vi "Setup For Triggered Images USB3 v4.4.vi"(5 "error in":errorcluster caption="error in (no error)", 6 "Timeout":u32=20000, 7 "Gain":dbl, 8 "Shutter speed":dbl=30000.0, 9 "Camera Name":T3="FL3-32S2M") -> (0 "Error out":errorcluster caption="error in (no error)", 1 "Session Out":T3="FL3-32S2M", 2 "Height":u32=1552, 3 "Width":u32=2080, 4 "DeviceID":string="FL3-32S2M")   [LabVIEW 2013]
doc: "The Grab and Attributes Setup VI acquires images continuously and displays the images in an image control using high-level acquisition VIs. The VI also modifes the camera attributes while acquiring images. A grab is appropriate for high-speed applications in which you need to process only one image at a time."
uses:
  <vilib>/userdefined/High Color/IMAQdx.ctl
  <vilib>/vision/driver/IMAQdx.llb/IMAQdx Attribute Type.ctl
  <vilib>/vision/driver/IMAQdx.llb/IMAQdx Attribute Visibility.ctl
  <vilib>/vision/driver/NI_Vision_Acquisition_Software.lvlib
  <resource>/objmgr/imaqdx.rc
panel:
  in  "stop":bool
  out "Attribute Information Array":T2(array[cluster])=[{"Attribute Type"=enum."U32", "Readable"=TRUE, "Writable"=TRUE, "Attribute Name"="AcquisitionAttributes::AdvancedGenicam::CommandTimeout"}, {"Attribute Type"=enum."U32", "Readable"=TRUE, "Writable"=TRUE, "Attribute Name"="AcquisitionAttributes::AdvancedGenicam::EventQueueDepth"}, {"Attribute Type"=enum."Bool", "Readable"=TRUE, "Writable"=FALSE, "Attribute Name"="AcquisitionAttributes::AdvancedGenicam::EventsEnabled"}, {"Attribute Type"=enum."Bool", "Readable"=TRUE, "Writable"=FALSE, "Attribute Name"="AcquisitionAttributes::AdvancedGenicam::EventsSupported"}, {"Attribute Type"=enum."Bool", "Readable"=TRUE, "Writable"=TRUE, "Attribute Name"="AcquisitionAttributes::AdvancedGenicam::IgnoreCameraValidationErrors"}, {"Attribute Type"=enum."U32", "Readable"=TRUE, "Writable"=FALSE, "Attribute Name"="AcquisitionAttributes::AdvancedUSB3Vision::ActualMaximumPayloadTransferSize"}, {"Attribute Type"=enum."U32", "Readable"=TRUE, "Writable"=FALSE, "Attribute Name"="AcquisitionAttributes::AdvancedUSB3Vision::RequiredPayloadSizeAlignment"}, {"Attribute Type"=enum."Enum", "Readable"=TRUE, "Writable"=TRUE, "Attribute Name"="AcquisitionAttributes::Bayer::Algorithm"}, {"Attribute Type"=enum."DBL", "Readable"=TRUE, "Writable"=TRUE, "Attribute Name"="AcquisitionAttributes::Bayer::GainB"}, {"Attribute Type"=enum."DBL", "Readable"=TRUE, "Writable"=TRUE, "Attribute Name"="AcquisitionAttributes::Bayer::GainG"}, {"Attribute Type"=enum."DBL", "Readable"=TRUE, "Writable"=TRUE, "Attribute Name"="AcquisitionAttributes::Bayer::GainR"}, {"Attribute Type"=enum."Enum", "Readable"=TRUE, "Writable"=TRUE, "Attribute Name"="AcquisitionAttributes::Bayer::Pattern"}, {"Attribute Type"=enum."Bool", "Readable"=TRUE, "Writable"=TRUE, "Attribute Name"="AcquisitionAttributes::ChunkDataDecoding::ChunkDataDecodingEnabled"}, {"Attribute Type"=enum."U32", "Readable"=TRUE, "Writable"=TRUE, "Attribute Name"="AcquisitionAttributes::ChunkDataDecoding::MaximumChunkCopySize"}, {"Attribute Type"=enum."Enum", "Readable"=TRUE, "Writable"=TRUE, "Attribute Name"="CameraAttributes::AnalogControl::GainAuto"}, {"Attribute Type"=enum."DBL", "Readable"=TRUE, "Writable"=TRUE, "Attribute Name"="CameraAttributes::AnalogControl::Gain"}, {"Attribute Type"=enum."DBL", "Readable"=TRUE, "Writable"=FALSE, "Attribute Name"="CameraAttributes::AnalogControl::AutoGainLowerLimit"}, {"Attribute Type"=enum."DBL", "Readable"=TRUE, "Writable"=FALSE, "Attribute Name"="CameraAttributes::AnalogControl::AutoGainUpperLimit"}, {"Attribute Type"=enum."DBL", "Readable"=TRUE, "Writable"=TRUE, "Attribute Name"="CameraAttributes::AnalogControl::BlackLevel"}, {"Attribute Type"=enum."Bool", "Readable"=TRUE, "Writable"=TRUE, "Attribute Name"="CameraAttributes::AnalogControl::BlackLevelEnabled"}, {"Attribute Type"=enum."DBL", "Readable"=TRUE, "Writable"=FALSE, "Attribute Name"="CameraAttributes::AnalogControl::Gamma"}, {"Attribute Type"=enum."Bool", "Readable"=TRUE, "Writable"=TRUE, "Attribute Name"="CameraAttributes::AnalogControl::GammaEnabled"}, {"Attribute Type"=enum."I64", "Readable"=TRUE, "Writable"=FALSE, "Attribute Name"="CameraAttributes::AnalogControl::Sharpness"}, {"Attribute Type"=enum."Bool", "Readable"=TRUE, "Writable"=TRUE, "Attribute Name"="CameraAttributes::AnalogControl::SharpnessEnabled"}, {"Attribute Type"=enum."Enum", "Readable"=TRUE, "Writable"=FALSE, "Attribute Name"="CameraAttributes::AnalogControl::SharpnessAuto"}, {"Attribute Type"=enum."Bool", "Readable"=FALSE, "Writable"=FALSE, "Attribute Name"="CameraAttributes::AnalogControl::HueEnabled"}, {"Attribute Type"=enum."Bool", "Readable"=FALSE, "Writable"=FALSE, "Attribute Name"="CameraAttributes::AnalogControl::SaturationEnabled"}, {"Attribute Type"=enum."String", "Readable"=TRUE, "Writable"=FALSE, "Attribute Name"="CameraAttributes::DeviceControl::DeviceVendorName"}, {"Attribute Type"=enum."String", "Readable"=TRUE, "Writable"=FALSE, "Attribute Name"="CameraAttributes::DeviceControl::DeviceModelName"}, {"Attribute Type"=enum."String", "Readable"=TRUE, "Writable"=FALSE, "Attribute Name"="CameraAttributes::DeviceControl::DeviceFamilyName"}, {"Attribute Type"=enum."String", "Readable"=TRUE, "Writable"=FALSE, "Attribute Name"="CameraAttributes::DeviceControl::DeviceVersion"}, {"Attribute Type"=enum."String", "Readable"=TRUE, "Writable"=FALSE, "Attribute Name"="CameraAttributes::DeviceControl::DeviceSVNVersion"}, {"Attribute Type"=enum."String", "Readable"=TRUE, "Writable"=FALSE, "Attribute Name"="CameraAttributes::DeviceControl::DeviceID"}, {"Attribute Type"=enum."String", "Readable"=TRUE, "Writable"=TRUE, "Attribute Name"="CameraAttributes::DeviceControl::DeviceUserID"}, {"Attribute Type"=enum."Enum", "Readable"=TRUE, "Writable"=FALSE, "Attribute Name"="CameraAttributes::DeviceControl::DeviceScanType"}, {"Attribute Type"=enum."DBL", "Readable"=TRUE, "Writable"=FALSE, "Attribute Name"="CameraAttributes::DeviceControl::DeviceTemperature"}, {"Attribute Type"=enum."I64", "Readable"=TRUE, "Writable"=FALSE, "Attribute Name"="CameraAttributes::DeviceControl::U3VDeviceCapability"}, {"Attribute Type"=enum."Bool", "Readable"=TRUE, "Writable"=FALSE, "Attribute Name"="CameraAttributes::DeviceControl::UserNameAvailable"}, {"Attribute Type"=enum."Bool", "Readable"=TRUE, "Writable"=FALSE, "Attribute Name"="CameraAttributes::DeviceControl::AccessPrivilegeAvailable"}, {"Attribute Type"=enum."Bool", "Readable"=TRUE, "Writable"=FALSE, "Attribute Name"="CameraAttributes::DeviceControl::MessageChannelSupported"}, {"Attribute Type"=enum."Bool", "Readable"=TRUE, "Writable"=FALSE, "Attribute Name"="CameraAttributes::DeviceControl::TimestampSupported"}, {"Attribute Type"=enum."I64", "Readable"=TRUE, "Writable"=FALSE, "Attribute Name"="CameraAttributes::DeviceControl::StringEncoding"}, {"Attribute Type"=enum."Bool", "Readable"=TRUE, "Writable"=FALSE, "Attribute Name"="CameraAttributes::DeviceControl::FamilyRegisterAvailable"}, {"Attribute Type"=enum."Bool", "Readable"=TRUE, "Writable"=FALSE, "Attribute Name"="CameraAttributes::DeviceControl::SBRMSupported"}, {"Attribute Type"=enum."Bool", "Readable"=TRUE, "Writable"=FALSE, "Attribute Name"="CameraAttributes::DeviceControl::EndianessRegistersSupported"}, {"Attribute Type"=enum."Bool", "Readable"=TRUE, "Writable"=FALSE, "Attribute Name"="CameraAttributes::DeviceControl::WrittenLengthFieldSupported"}, {"Attribute Type"=enum."I64", "Readable"=TRUE, "Writable"=FALSE, "Attribute Name"="CameraAttributes::DeviceControl::DeviceMaxThroughput"}, {"Attribute Type"=enum."I64", "Readable"=TRUE, "Writable"=TRUE, "Attribute Name"="CameraAttributes::DeviceControl::DeviceLinkThroughputLimit"}, {"Attribute Type"=enum."Enum", "Readable"=TRUE, "Writable"=TRUE, "Attribute Name"="CameraAttributes::AcquisitionControl::TriggerSelector"}, {"Attribute Type"=enum."Enum", "Readable"=TRUE, "Writable"=TRUE, "Attribute Name"="CameraAttributes::AcquisitionControl::TriggerMode"}, {"Attribute Type"=enum."Command", "Readable"=FALSE, "Writable"=FALSE, "Attribute Name"="CameraAttributes::AcquisitionControl::TriggerSoftware"}, {"Attribute Type"=enum."Enum", "Readable"=TRUE, "Writable"=TRUE, "Attribute Name"="CameraAttributes::AcquisitionControl::TriggerSource"}, {"Attribute Type"=enum."Enum", "Readable"=TRUE, "Writable"=TRUE, "Attribute Name"="CameraAttributes::AcquisitionControl::TriggerActivation"}, {"Attribute Type"=enum."DBL", "Readable"=TRUE, "Writable"=TRUE, "Attribute Name"="CameraAttributes::AcquisitionControl::TriggerDelay"}, {"Attribute Type"=enum."Bool", "Readable"=TRUE, "Writable"=TRUE, "Attribute Name"="CameraAttributes::AcquisitionControl::TriggerDelayEnabled"}, {"Attribute Type"=enum."Enum", "Readable"=TRUE, "Writable"=TRUE, "Attribute Name"="CameraAttributes::AcquisitionControl::ExposureMode"}, {"Attribute Type"=enum."Enum", "Readable"=TRUE, "Writable"=TRUE, "Attribute Name"="CameraAttributes::AcquisitionControl::ExposureAuto"}, {"Attribute Type"=enum."DBL", "Readable"=TRUE, "Writable"=FALSE, "Attribute Name"="CameraAttributes::AcquisitionControl::ExposureTime"}, {"Attribute Type"=enum."DBL", "Readable"=TRUE, "Writable"=TRUE, "Attribute Name"="CameraAttributes::AcquisitionControl::AutoExposureTimeLowerLimit"}, {"Attribute Type"=enum."DBL", "Readable"=TRUE, "Writable"=TRUE, "Attribute Name"="CameraAttributes::AcquisitionControl::AutoExposureTimeUpperLimit"}, {"Attribute Type"=enum."Enum", "Readable"=TRUE, "Writable"=TRUE, "Attribute Name"="CameraAttributes::AcquisitionControl::AcquisitionMode"}, {"Attribute Type"=enum."Enum", "Readable"=TRUE, "Writable"=TRUE, "Attribute Name"="CameraAttributes::AcquisitionControl::AcquisitionFrameRateAuto"}, {"Attribute Type"=enum."Bool", "Readable"=TRUE, "Writable"=TRUE, "Attribute Name"="CameraAttributes::AcquisitionControl::AcquisitionFrameRateEnabled"}, {"Attribute Type"=enum."DBL", "Readable"=TRUE, "Writable"=FALSE, "Attribute Name"="CameraAttributes::AcquisitionControl::AcquisitionFrameRate"}, {"Attribute Type"=enum."I64", "Readable"=FALSE, "Writable"=FALSE, "Attribute Name"="CameraAttributes::AcquisitionControl::AcquisitionFrameCount"}, {"Attribute Type"=enum."Enum", "Readable"=TRUE, "Writable"=TRUE, "Attribute Name"="CameraAttributes::ImageFormatControl::PixelFormat"}, {"Attribute Type"=enum."I64", "Readable"=TRUE, "Writable"=TRUE, "Attribute Name"="CameraAttributes::ImageFormatControl::Width"}, {"Attribute Type"=enum."I64", "Readable"=TRUE, "Writable"=TRUE, "Attribute Name"="CameraAttributes::ImageFormatControl::Height"}, {"Attribute Type"=enum."I64", "Readable"=TRUE, "Writable"=TRUE, "Attribute Name"="CameraAttributes::ImageFormatControl::OffsetX"}, {"Attribute Type"=enum."I64", "Readable"=TRUE, "Writable"=TRUE, "Attribute Name"="CameraAttributes::ImageFormatControl::OffsetY"}, {"Attribute Type"=enum."I64", "Readable"=TRUE, "Writable"=FALSE, "Attribute Name"="CameraAttributes::ImageFormatControl::SensorWidth"}, {"Attribute Type"=enum."I64", "Readable"=TRUE, "Writable"=FALSE, "Attribute Name"="CameraAttributes::ImageFormatControl::SensorHeight"}, {"Attribute Type"=enum."I64", "Readable"=TRUE, "Writable"=FALSE, "Attribute Name"="CameraAttributes::ImageFormatControl::WidthMax"}, {"Attribute Type"=enum."I64", "Readable"=TRUE, "Writable"=FALSE, "Attribute Name"="CameraAttributes::ImageFormatControl::HeightMax"}, {"Attribute Type"=enum."Enum", "Readable"=TRUE, "Writable"=TRUE, "Attribute Name"="CameraAttributes::ImageFormatControl::VideoMode"}, {"Attribute Type"=enum."I64", "Readable"=TRUE, "Writable"=FALSE, "Attribute Name"="CameraAttributes::ImageFormatControl::BinningHorizontal"}, {"Attribute Type"=enum."I64", "Readable"=TRUE, "Writable"=TRUE, "Attribute Name"="CameraAttributes::ImageFormatControl::BinningVertical"}, {"Attribute Type"=enum."Bool", "Readable"=TRUE, "Writable"=TRUE, "Attribute Name"="CameraAttributes::ImageFormatControl::ReverseX"}, {"Attribute Type"=enum."Enum", "Readable"=TRUE, "Writable"=FALSE, "Attribute Name"="CameraAttributes::ImageFormatControl::PixelCoding"}, {"Attribute Type"=enum."Enum", "Readable"=TRUE, "Writable"=FALSE, "Attribute Name"="CameraAttributes::ImageFormatControl::PixelSize"}, {"Attribute Type"=enum."Enum", "Readable"=TRUE, "Writable"=FALSE, "Attribute Name"="CameraAttributes::ImageFormatControl::PixelColorFilter"}, {"Attribute Type"=enum."I64", "Readable"=TRUE, "Writable"=FALSE, "Attribute Name"="CameraAttributes::ImageFormatControl::PixelDynamicRangeMin"}, {"Attribute Type"=enum."I64", "Readable"=TRUE, "Writable"=FALSE, "Attribute Name"="CameraAttributes::ImageFormatControl::PixelDynamicRangeMax"}, {"Attribute Type"=enum."Enum", "Readable"=TRUE, "Writable"=TRUE, "Attribute Name"="CameraAttributes::ImageFormatControl::TestImageSelector"}, {"Attribute Type"=enum."I64", "Readable"=TRUE, "Writable"=FALSE, "Attribute Name"="CameraAttributes::UserSetControl::UserSetCurrent"}, {"Attribute Type"=enum."Enum", "Readable"=TRUE, "Writable"=TRUE, "Attribute Name"="CameraAttributes::UserSetControl::UserSetSelector"}, {"Attribute Type"=enum."Enum", "Readable"=TRUE, "Writable"=TRUE, "Attribute Name"="CameraAttributes::UserSetControl::UserSetDefaultSelector"}, {"Attribute Type"=enum."Command", "Readable"=FALSE, "Writable"=TRUE, "Attribute Name"="CameraAttributes::UserSetControl::UserSetLoad"}, {"Attribute Type"=enum."Command", "Readable"=FALSE, "Writable"=TRUE, "Attribute Name"="CameraAttributes::UserSetControl::UserSetSave"}, {"Attribute Type"=enum."Enum", "Readable"=TRUE, "Writable"=TRUE, "Attribute Name"="CameraAttributes::DigitalIOControl::LineSelector"}, {"Attribute Type"=enum."Enum", "Readable"=TRUE, "Writable"=TRUE, "Attribute Name"="CameraAttributes::DigitalIOControl::LineMode"}, {"Attribute Type"=enum."Enum", "Readable"=FALSE, "Writable"=FALSE, "Attribute Name"="CameraAttributes::DigitalIOControl::LineSource"}, {"Attribute Type"=enum."Bool", "Readable"=FALSE, "Writable"=FALSE, "Attribute Name"="CameraAttributes::DigitalIOControl::LineInverter"}, {"Attribute Type"=enum."I64", "Readable"=TRUE, "Writable"=TRUE, "Attribute Name"="CameraAttributes::DigitalIOControl::LineDebouncerTimeRaw"}, {"Attribute Type"=enum."Bool", "Readable"=TRUE, "Writable"=FALSE, "Attribute Name"="CameraAttributes::DigitalIOControl::LineStatus"}, {"Attribute Type"=enum."I64", "Readable"=TRUE, "Writable"=FALSE, "Attribute Name"="CameraAttributes::DigitalIOControl::LineStatusAll"}, {"Attribute Type"=enum."Bool", "Readable"=FALSE, "Writable"=FALSE, "Attribute Name"="CameraAttributes::DigitalIOControl::StrobeEnabled"}, {"Attribute Type"=enum."DBL", "Readable"=FALSE, "Writable"=FALSE, "Attribute Name"="CameraAttributes::DigitalIOControl::StrobeDelay"}, {"Attribute Type"=enum."DBL", "Readable"=FALSE, "Writable"=FALSE, "Attribute Name"="CameraAttributes::DigitalIOControl::StrobeDuration"}, {"Attribute Type"=enum."Bool", "Readable"=FALSE, "Writable"=FALSE, "Attribute Name"="CameraAttributes::DigitalIOControl::UserOutputValue"}, {"Attribute Type"=enum."I64", "Readable"=TRUE, "Writable"=FALSE, "Attribute Name"="CameraAttributes::TransportLayerControl::PayloadSize"}, {"Attribute Type"=enum."I64", "Readable"=TRUE, "Writable"=FALSE, "Attribute Name"="CameraAttributes::TransportLayerControl::GenCPVersionMajor"}, {"Attribute Type"=enum."I64", "Readable"=TRUE, "Writable"=FALSE, "Attribute Name"="CameraAttributes::TransportLayerControl::GenCPVersionMinor"}, {"Attribute Type"=enum."I64", "Readable"=TRUE, "Writable"=FALSE, "Attribute Name"="CameraAttributes::TransportLayerControl::U3VTimestamp"}, {"Attribute Type"=enum."Command", "Readable"=FALSE, "Writable"=TRUE, "Attribute Name"="CameraAttributes::TransportLayerControl::U3VTimestampLatch"}, {"Attribute Type"=enum."I64", "Readable"=TRUE, "Writable"=FALSE, "Attribute Name"="CameraAttributes::TransportLayerControl::U3VTimestampIncrement"}, {"Attribute Type"=enum."I64", "Readable"=TRUE, "Writable"=FALSE, "Attribute Name"="CameraAttributes::TransportLayerControl::U3VVersionMajor"}, {"Attribute Type"=enum."I64", "Readable"=TRUE, "Writable"=FALSE, "Attribute Name"="CameraAttributes::TransportLayerControl::U3VVersionMinor"}, {"Attribute Type"=enum."I64", "Readable"=TRUE, "Writable"=FALSE, "Attribute Name"="CameraAttributes::TransportLayerControl::U3VCPCapability"}, {"Attribute Type"=enum."Bool", "Readable"=TRUE, "Writable"=FALSE, "Attribute Name"="CameraAttributes::TransportLayerControl::U3VCPSIRMAvailable"}, {"Attribute Type"=enum."Bool", "Readable"=TRUE, "Writable"=FALSE, "Attribute Name"="CameraAttributes::TransportLayerControl::U3VCPEIRMAvailable"}, {"Attribute Type"=enum."Bool", "Readable"=TRUE, "Writable"=FALSE, "Attribute Name"="CameraAttributes::TransportLayerControl::U3VCPIIDC2Available"}, {"Attribute Type"=enum."I64", "Readable"=TRUE, "Writable"=FALSE, "Attribute Name"="CameraAttributes::TransportLayerControl::U3VMaxCommandTransferLength"}, {"Attribute Type"=enum."I64", "Readable"=TRUE, "Writable"=FALSE, "Attribute Name"="CameraAttributes::TransportLayerControl::U3VMaxAcknowledgeTransferLength"}, {"Attribute Type"=enum."I64", "Readable"=TRUE, "Writable"=FALSE, "Attribute Name"="CameraAttributes::TransportLayerControl::U3VNumberOfStreamChannels"}, {"Attribute Type"=enum."Enum", "Readable"=TRUE, "Writable"=FALSE, "Attribute Name"="CameraAttributes::TransportLayerControl::U3VCurrentSpeed"}, {"Attribute Type"=enum."Bool", "Readable"=TRUE, "Writable"=TRUE, "Attribute Name"="CameraAttributes::ChunkDataControl::ChunkModeActive"}, {"Attribute Type"=enum."Enum", "Readable"=TRUE, "Writable"=TRUE, "Attribute Name"="CameraAttributes::ChunkDataControl::ChunkSelector"}, {"Attribute Type"=enum."Bool", "Readable"=TRUE, "Writable"=TRUE, "Attribute Name"="CameraAttributes::ChunkDataControl::ChunkEnable"}, {"Attribute Type"=enum."I64", "Readable"=FALSE, "Writable"=FALSE, "Attribute Name"="CameraAttributes::ChunkDataControl::ChunkImage"}, {"Attribute Type"=enum."I64", "Readable"=FALSE, "Writable"=FALSE, "Attribute Name"="CameraAttributes::ChunkDataControl::ChunkCRC"}, {"Attribute Type"=enum."I64", "Readable"=FALSE, "Writable"=FALSE, "Attribute Name"="CameraAttributes::ChunkDataControl::ChunkFrameCounter"}, {"Attribute Type"=enum."I64", "Readable"=FALSE, "Writable"=FALSE, "Attribute Name"="CameraAttributes::ChunkDataControl::ChunkOffsetX"}, {"Attribute Type"=enum."I64", "Readable"=FALSE, "Writable"=FALSE, "Attribute Name"="CameraAttributes::ChunkDataControl::ChunkOffsetY"}, {"Attribute Type"=enum."I64", "Readable"=FALSE, "Writable"=FALSE, "Attribute Name"="CameraAttributes::ChunkDataControl::ChunkWidth"}, {"Attribute Type"=enum."I64", "Readable"=FALSE, "Writable"=FALSE, "Attribute Name"="CameraAttributes::ChunkDataControl::ChunkHeight"}, {"Attribute Type"=enum."DBL", "Readable"=FALSE, "Writable"=FALSE, "Attribute Name"="CameraAttributes::ChunkDataControl::ChunkExposureTime"}, {"Attribute Type"=enum."DBL", "Readable"=FALSE, "Writable"=FALSE, "Attribute Name"="CameraAttributes::ChunkDataControl::ChunkGain"}, {"Attribute Type"=enum."DBL", "Readable"=FALSE, "Writable"=FALSE, "Attribute Name"="CameraAttributes::ChunkDataControl::ChunkBlackLevel"}, {"Attribute Type"=enum."Enum", "Readable"=TRUE, "Writable"=TRUE, "Attribute Name"="AcquisitionAttributes::BitsPerPixel"}, {"Attribute Type"=enum."Enum", "Readable"=TRUE, "Writable"=TRUE, "Attribute Name"="AcquisitionAttributes::ImageDecoderCopyMode"}, {"Attribute Type"=enum."Enum", "Readable"=TRUE, "Writable"=TRUE, "Attribute Name"="AcquisitionAttributes::IncompleteBufferMode"}, {"Attribute Type"=enum."Enum", "Readable"=TRUE, "Writable"=TRUE, "Attribute Name"="AcquisitionAttributes::OutputImageType"}, {"Attribute Type"=enum."Enum", "Readable"=TRUE, "Writable"=TRUE, "Attribute Name"="AcquisitionAttributes::OverwriteMode"}, {"Attribute Type"=enum."Enum", "Readable"=TRUE, "Writable"=TRUE, "Attribute Name"="AcquisitionAttributes::ReceiveTimestampMode"}, {"Attribute Type"=enum."Bool", "Readable"=TRUE, "Writable"=TRUE, "Attribute Name"="AcquisitionAttributes::ShiftPixelBits"}, {"Attribute Type"=enum."Bool", "Readable"=TRUE, "Writable"=TRUE, "Attribute Name"="AcquisitionAttributes::SwapPixelBytes"}, {"Attribute Type"=enum."U32", "Readable"=TRUE, "Writable"=TRUE, "Attribute Name"="AcquisitionAttributes::Timeout"}, {"Attribute Type"=enum."U32", "Readable"=TRUE, "Writable"=FALSE, "Attribute Name"="CameraInformation::BaseAddress"}, {"Attribute Type"=enum."Enum", "Readable"=TRUE, "Writable"=FALSE, "Attribute Name"="CameraInformation::BusType"}, {"Attribute Type"=enum."String", "Readable"=TRUE, "Writable"=FALSE, "Attribute Name"="CameraInformation::ModelName"}, {"Attribute Type"=enum."String", "Readable"=TRUE, "Writable"=FALSE, "Attribute Name"="CameraInformation::PrimaryURLString"}, {"Attribute Type"=enum."String", "Readable"=TRUE, "Writable"=FALSE, "Attribute Name"="CameraInformation::SecondaryURLString"}, {"Attribute Type"=enum."U32", "Readable"=TRUE, "Writable"=FALSE, "Attribute Name"="CameraInformation::SerialNumberHigh"}, {"Attribute Type"=enum."U32", "Readable"=TRUE, "Writable"=FALSE, "Attribute Name"="CameraInformation::SerialNumberLow"}, {"Attribute Type"=enum."Enum", "Readable"=TRUE, "Writable"=FALSE, "Attribute Name"="CameraInformation::USBConnectionSpeed"}, {"Attribute Type"=enum."String", "Readable"=TRUE, "Writable"=FALSE, "Attribute Name"="CameraInformation::VendorName"}, {"Attribute Type"=enum."Bool", "Readable"=TRUE, "Writable"=FALSE, "Attribute Name"="StatusInformation::AcqInProgress"}, {"Attribute Type"=enum."I64", "Readable"=TRUE, "Writable"=FALSE, "Attribute Name"="StatusInformation::HandledEventCount"}, {"Attribute Type"=enum."I64", "Readable"=TRUE, "Writable"=FALSE, "Attribute Name"="StatusInformation::IncompleteBufferCount"}, {"Attribute Type"=enum."I64", "Readable"=TRUE, "Writable"=FALSE, "Attribute Name"="StatusInformation::LastBufferCount"}, {"Attribute Type"=enum."U32", "Readable"=TRUE, "Writable"=FALSE, "Attribute Name"="StatusInformation::LastBufferNumber"}, {"Attribute Type"=enum."I64", "Readable"=TRUE, "Writable"=FALSE, "Attribute Name"="StatusInformation::LostBufferCount"}, {"Attribute Type"=enum."I64", "Readable"=TRUE, "Writable"=FALSE, "Attribute Name"="StatusInformation::LostEventCount"}]
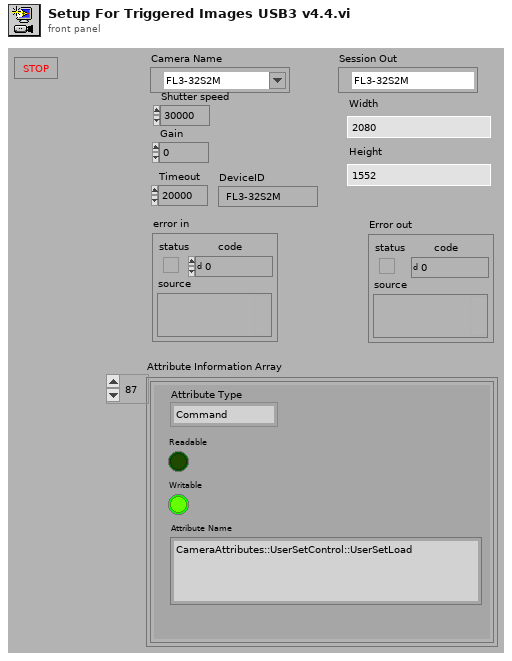
[diagram p1: front panel]
types:
  T1 = typedef "NI_Vision_Acquisition_Software.lvlib/IMAQdx Attribute Type.ctl" = enum32{"U32", "I64", "DBL", "String", "Enum", "Bool", "Command"}
  T2 = cluster{"Attribute Type":T1, "Readable":bool, "Writable":bool, "Attribute Name":string}[]
  T3 = typedef "IMAQdx.ctl" = refnum<k21>
  T4 = typedef "NI_Vision_Acquisition_Software.lvlib/IMAQdx Attribute Visibility.ctl" = enum32{"Simple", "Intermediate", "Advanced"}
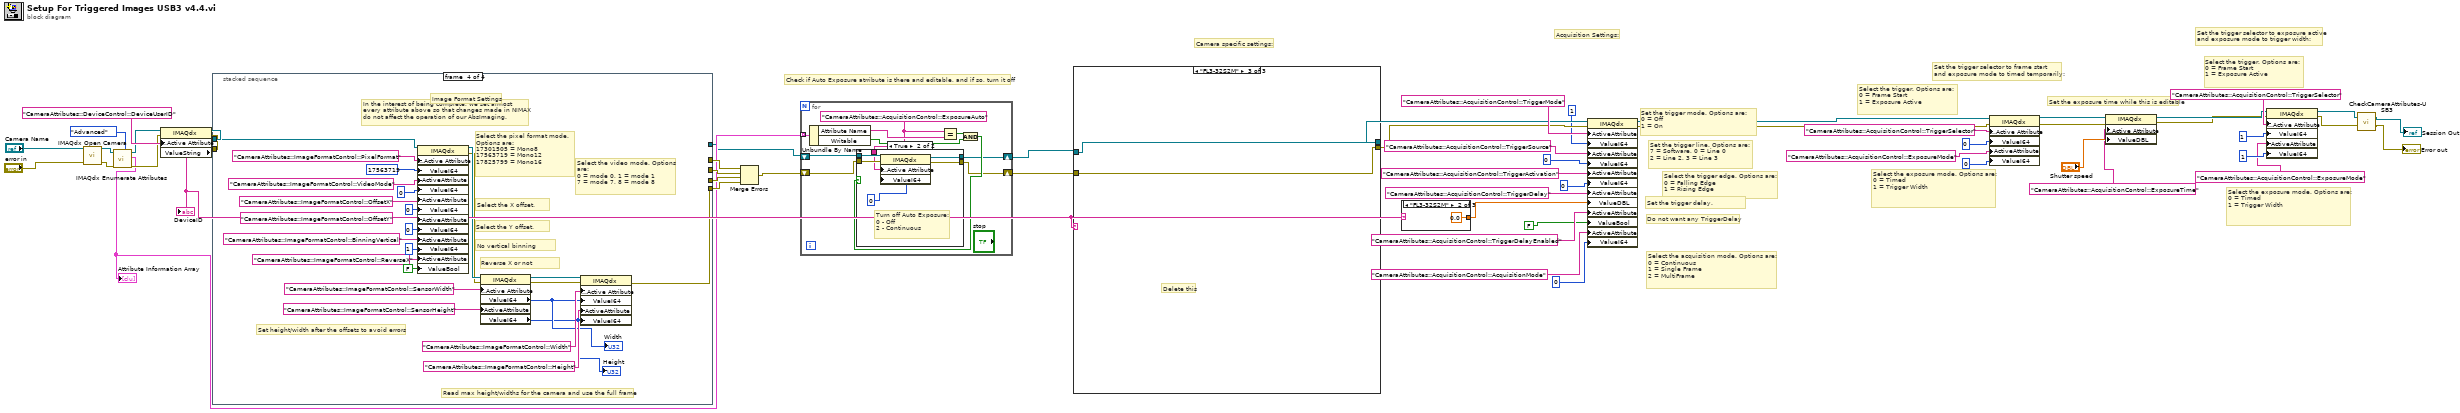
[diagram p0: block diagram]
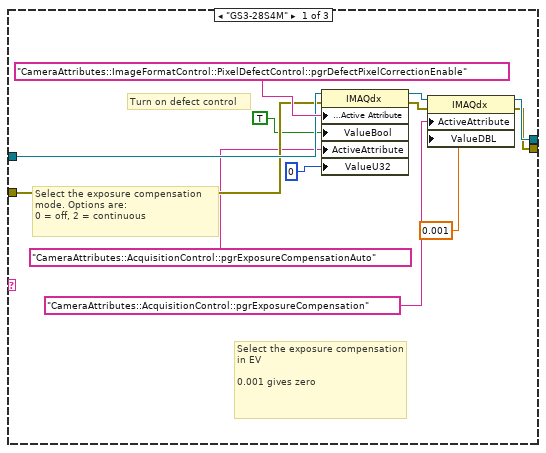
[diagram p3: hidden frame]
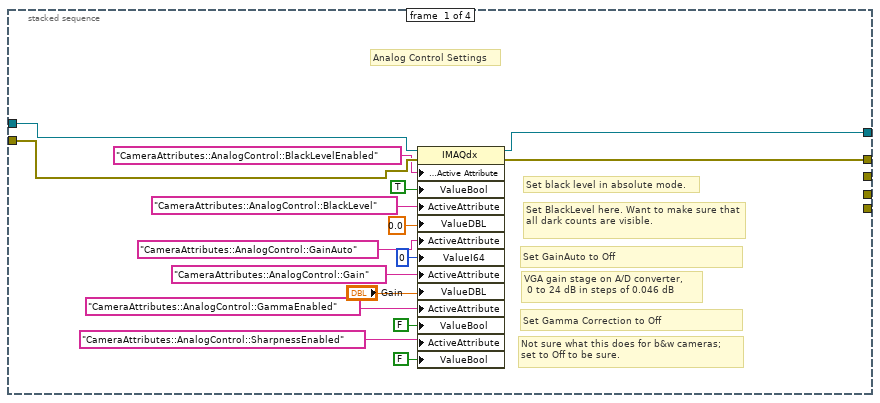
[diagram p5: hidden frame]
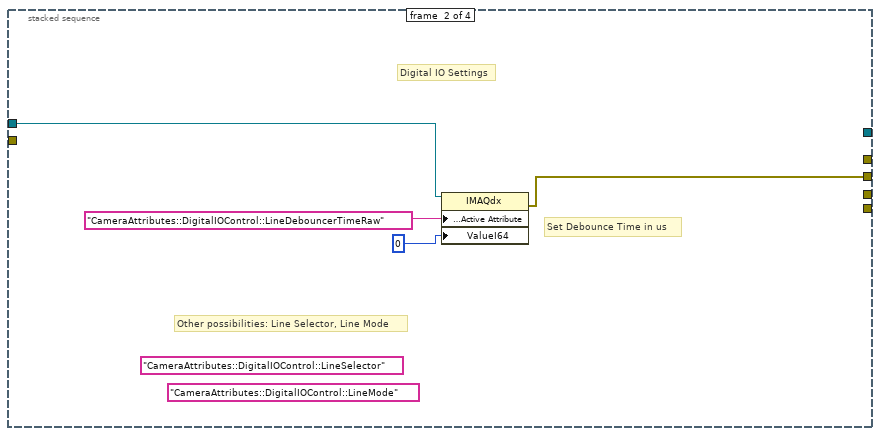
[diagram p6: hidden frame]
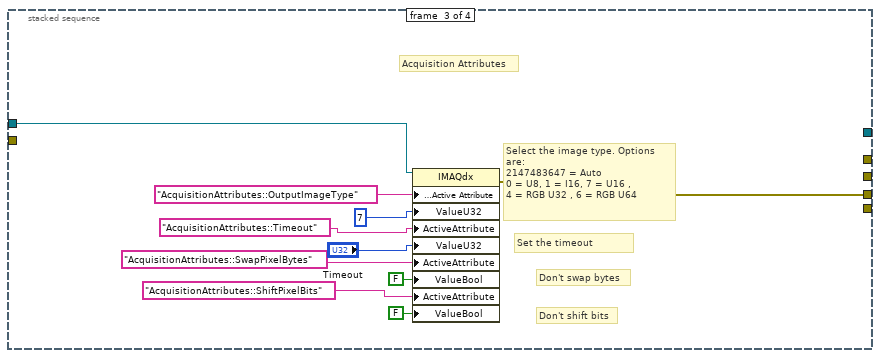
[diagram p7: hidden frame]
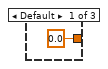
[diagram p8: hidden frame]
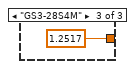
[diagram p9: hidden frame]
diagram:
  # "Acquisition Settings:"
  # "Camera specific settings:"
  # "Check if Auto Exposure atrribute is there and editable, and if so, turn it off"
  # "Set the exposure time while this is editable"
  # "Set the trigger selector to exposure active\nand exposure mode to trigger width:"
  # "Select the exposure mode. Options are:\n0 = Timed\n1 = Trigger Width"
  # "Select the trigger. Options are:\n0 = Frame Start\n1 = Exposure Active"
  # "Set the trigger selector to frame start \nand exposure mode to timed temporarily:"
  # "Do not want any TriggerDelay"
  # "Select the acquisition mode. Options are:\n0 = Continuous\n1 = Single Frame\n2 = MultiFrame"
  # "Select the exposure mode. Options are:\n0 = Timed\n1 = Trigger Width"
  # "Select the trigger edge. Options are:\n0 = Falling Edge\n1 = Rising Edge"
  # "Select the trigger. Options are:\n0 = Frame Start\n1 = Exposure Active"
  # "Set the trigger mode. Options are:\n0 = Off\n1 = On"
  # "Set the trigger delay."
  # "Set the trigger line. Options are:\n7 = Software, 0 = Line 0\n2 = Line 2, 3 = Line 3"
  # "In the interest of being complete, we set almost\nevery attribute above so that changes made in NIMAX\ndo not affect the operation of our AbsImaging."
  n1 = call <vilib>:"IMAQdx Open Camera.vi"("error in"="error in", "Session In"="Camera Name") -> ("error out"=w49:errorcluster, "Session Out"=w51:T3)  [unwired: 1 in, 7 out]
  n2 = call <vilib>:"IMAQdx Enumerate Attributes.vi"("Visibility"=IMAQdx_Attribute_Visibility."Advanced", "error in"=w49, "Session In"=w51) -> ("error out"=w48:errorcluster, "Attribute Information Array"=w9:T2, "Session Out"=w47:T3)  [unwired: 1 in, 5 out]
  "Attribute Information Array" <- w9
  n3 = property class="IMAQdx"(reference=w47, error in=w48, "Camera Attributes:Active Attribute"="CameraAttributes::DeviceControl::DeviceUserID" ("ActiveAttribute")) -> (reference out=w46:T3, error out=w45:errorcluster, "ValueString"=w10:string)
  "DeviceID" <- w10
  n4 = stacked-sequence {
    tunnel: w46 -> [w61 w72 w84 w108]
    tunnel: w45 -> [w60 _ _ _]
    tunnel: [w56 _ _ _] -> w14
    tunnel: [_ w71 _ _] -> w13
    tunnel: [_ _ w83 _] -> w12
    tunnel: [w55 _ _ _] -> w8
    tunnel: [_ _ _ w89] -> w11
    frame #0 {
      # "Analog Control Settings"
      # "Not sure what this does for b&w cameras;\nset to Off to be sure."
      # "Set Gamma Correction to Off"
      # "VGA gain stage on A/D converter,\n 0 to 24 dB in steps of 0.046 dB"
      # "Set GainAuto to Off"
      # "Set BlackLevel here. Want to make sure that all dark counts are visible."
      # "Set black level in absolute mode."
      n5 = property class="IMAQdx"(reference=w61, error in=w60, "Camera Attributes:Active Attribute"="CameraAttributes::AnalogControl::BlackLevelEnabled" ("ActiveAttribute"), "ValueBool"=TRUE, "ActiveAttribute"="CameraAttributes::AnalogControl::BlackLevel", "ValueDBL"=0.0, "ActiveAttribute"="CameraAttributes::AnalogControl::GainAuto", "ValueI64"=i64 0, "ActiveAttribute"="CameraAttributes::AnalogControl::Gain", "ValueDBL"="Gain", "ActiveAttribute"="CameraAttributes::AnalogControl::GammaEnabled", "ValueBool"=FALSE, "ActiveAttribute"="CameraAttributes::AnalogControl::SharpnessEnabled", "ValueBool"=FALSE) -> (reference out=w55:T3, error out=w56:errorcluster)
    }
    frame #1 {
      (unwired) "CameraAttributes::DigitalIOControl::LineMode" ("ActiveAttribute")
      (unwired) "CameraAttributes::DigitalIOControl::LineSelector" ("ActiveAttribute")
      # "Digital IO Settings"
      # "Other possibilities: Line Selector, Line Mode"
      # "Set Debounce Time in us"
      n6 = property class="IMAQdx"(reference=w72, "Camera Attributes:Active Attribute"="CameraAttributes::DigitalIOControl::LineDebouncerTimeRaw" ("ActiveAttribute"), "ValueI64"=i64 0) -> (error out=w71:errorcluster)  [unwired: 1 in, 1 out]
    }
    frame #2 {
      # "Acquisition Attributes"
      # "Don't swap bytes"
      # "Don't shift bits"
      # "Set the timeout"
      # "Select the image type. Options are:\n2147483647 = Auto\n0 = U8, 1 = I16, 7 = U16 , \n4 = RGB U32 , 6 = RGB U64"
      n7 = property class="IMAQdx"(reference=w84, "Camera Attributes:Active Attribute"="AcquisitionAttributes::OutputImageType" ("ActiveAttribute"), "ValueU32"=i64 7 ("ValueI64"), "ActiveAttribute"="AcquisitionAttributes::Timeout", "ValueU32"="Timeout", "ActiveAttribute"="AcquisitionAttributes::SwapPixelBytes", "ValueBool"=FALSE, "ActiveAttribute"="AcquisitionAttributes::ShiftPixelBits", "ValueBool"=FALSE) -> (error out=w83:errorcluster)  [unwired: 1 in, 1 out]
    }
    frame #3 {
      # "Image Format Settings"
      # "Reverse X or not"
      # "Read max height/widths for the camera and use the full frame"
      # "Set height/width after the offsets to avoid errors"
      # "No vertical binning"
      # "Select the X offset."
      # "Select the Y offset."
      # "Select the video mode. Options are:\n0 = mode 0, 1 = mode 1\n7 = mode 7, 8 = mode 8"
      # "Select the pixel format mode. Options are:\n17301505 = Mono8\n17563719 = Mono12\n17825799 = Mono16"
      n8 = property class="IMAQdx"(reference=w108, "Camera Attributes:Active Attribute"="CameraAttributes::ImageFormatControl::PixelFormat" ("ActiveAttribute"), "ValueI64"=i64 17563719, "ActiveAttribute"="CameraAttributes::ImageFormatControl::VideoMode", "ValueI64"=i64 0, "ActiveAttribute"="CameraAttributes::ImageFormatControl::OffsetX", "ValueI64"=i64 0, "ActiveAttribute"="CameraAttributes::ImageFormatControl::OffsetY", "ValueI64"=i64 0, "ActiveAttribute"="CameraAttributes::ImageFormatControl::BinningVertical", "ValueI64"=i64 1, "ActiveAttribute"="CameraAttributes::ImageFormatControl::ReverseX", "ValueBool"=FALSE) -> (reference out=w97:T3, error out=w96:errorcluster)  [unwired: 1 in]
      n9 = property class="IMAQdx"(reference=w97, error in=w96, "Camera Attributes:Active Attribute"="CameraAttributes::ImageFormatControl::SensorWidth" ("ActiveAttribute"), "ActiveAttribute"="CameraAttributes::ImageFormatControl::SensorHeight") -> (reference out=w91:T3, error out=w90:errorcluster, "ValueI64"=w88:i64, "ValueI64"=w87:i64)
      "Width" <- w88
      "Height" <- w87
      n10 = property class="IMAQdx"(reference=w91, error in=w90, "Camera Attributes:Active Attribute"="CameraAttributes::ImageFormatControl::Width" ("ActiveAttribute"), "ValueI64"=w88, "ActiveAttribute"="CameraAttributes::ImageFormatControl::Height", "ValueI64"=w87) -> (error out=w89:errorcluster)  [unwired: 1 out]
    }
  }
  n11 = Merge Errors(w14, w13, w12, w11) -> (w7:errorcluster)
  n12 = for {
    tunnel: w9 -> [w118] mode=indexing
    shift-right: [w110] -> w6
    shift-left: w8 -> [w113]
    shift-right: [w109] -> w5
    shift-left: w7 -> [w112]
    w111 = "CameraAttributes::AcquisitionControl::ExposureAuto" ("ActiveAttribute")
    n13 = Unbundle By Name(w118) -> ("Attribute Name"=w117:string, "Writable"=w115:bool)
    n14 = Equal?(x=w111, y=w117) -> (x = y?=w116:bool)
    n15 = And(x=w116, y=w115) -> (x .and. y?=w114:bool)
    n16 = case shown="True" w114 {
      tunnel: w113 -> [w120 w125]
      tunnel: w112 -> [w119 w124]
      tunnel: [w120 w123] -> w110
      tunnel: [w119 w122] -> w109
      tunnel: w111 -> [_ w121]
      frame False {
      }
      frame True {
        # "Turn off Auto Exposure:\n0 - Off\n2 - Continuous"
        n17 = property class="IMAQdx"(reference=w125, error in=w124, "Camera Attributes:Active Attribute"=w121, "ValueI64"=i64 0) -> (reference out=w123:T3, error out=w122:errorcluster)
      }
    }
  }
  n18 = case shown="\"FL3-32S2M\"" w10 {
    tunnel: w6 -> [w137 w140 w142]
    tunnel: [w130 w140 w142] -> w35
    tunnel: [w129 w139 w141] -> w34
    tunnel: w5 -> [w136 w139 w141]
    frame "GS3-28S4M" {
      # "Select the exposure compensation in EV\n\n0.001 gives zero"
      # "Select the exposure compensation mode. Options are:\n0 = off, 2 = continuous"
      # "Turn on defect control"
      n19 = property class="IMAQdx"(reference=w137, error in=w136, "Camera Attributes:Active Attribute"="CameraAttributes::ImageFormatControl::PixelDefectControl::pgrDefectPixelCorrectionEnable" ("ActiveAttribute"), "ValueBool"=TRUE, "ActiveAttribute"="CameraAttributes::AcquisitionControl::pgrExposureCompensationAuto", "ValueU32"=u32 0) -> (reference out=w132:T3, error out=w131:errorcluster)
      n20 = property class="IMAQdx"(reference=w132, error in=w131, "ActiveAttribute"="CameraAttributes::AcquisitionControl::pgrExposureCompensation", "ValueDBL"=0.001) -> (reference out=w130:T3, error out=w129:errorcluster)
    }
    frame Default {
    }
    frame "FL3-32S2M" {
      # "Delete this"
    }
  }
  n21 = case shown="\"FL3-32S2M\"" w10 {
    tunnel: [0.0 ("ValueDBL") 0.0 ("ValueDBL") 1.2517 ("ValueDBL")] -> w38
    frame Default {
    }
    frame "FL3-32S2M" {
    }
    frame "GS3-28S4M" {
    }
  }
  n22 = property class="IMAQdx"(reference=w35, error in=w34, "ActiveAttribute"="CameraAttributes::AcquisitionControl::TriggerMode", "ValueI64"=i64 1, "ActiveAttribute"="CameraAttributes::AcquisitionControl::TriggerSource", "ValueI64"=i64 0, "ActiveAttribute"="CameraAttributes::AcquisitionControl::TriggerActivation", "ValueI64"=i64 0, "ActiveAttribute"="CameraAttributes::AcquisitionControl::TriggerDelay", "ValueDBL"=w38, "ActiveAttribute"="CameraAttributes::AcquisitionControl::TriggerDelayEnabled", "ValueBool"=FALSE, "ActiveAttribute"="CameraAttributes::AcquisitionControl::AcquisitionMode", "ValueI64"=i64 0) -> (reference out=w33:T3, error out=w32:errorcluster)
  n23 = property class="IMAQdx"(reference=w33, error in=w32, "Camera Attributes:Active Attribute"="CameraAttributes::AcquisitionControl::TriggerSelector" ("ActiveAttribute"), "ValueI64"=i64 0, "ActiveAttribute"="CameraAttributes::AcquisitionControl::ExposureMode", "ValueI64"=i64 0) -> (reference out=w22:T3, error out=w23:errorcluster)
  n24 = property class="IMAQdx"(reference=w22, error in=w23, "Camera Attributes:Active Attribute"="CameraAttributes::AcquisitionControl::ExposureTime" ("ActiveAttribute"), "ValueDBL"="Shutter speed") -> (reference out=w18:T3, error out=w17:errorcluster)
  n25 = property class="IMAQdx"(reference=w18, error in=w17, "Camera Attributes:Active Attribute"="CameraAttributes::AcquisitionControl::TriggerSelector" ("ActiveAttribute"), "ValueI64"=i64 1, "ActiveAttribute"="CameraAttributes::AcquisitionControl::ExposureMode", "ValueI64"=i64 1) -> (reference out=w4:T3, error out=w3:errorcluster)
  n26 = call "CheckCameraAttributes-USB3.vi"("error in"=w3, "Camera Name"=w4) -> ("error out"=→"Error out":errorcluster, "Session Out"=→"Session Out":T3)
